vi "Append Block.vi"(10 "block in":u8[](array[numeric]) format="%02x", 11 "Hash Function in":refnum<class "NI_SHA-256.lvclass">) -> (3 "Hash Function out":refnum<class "NI_SHA-256.lvclass">)   [LabVIEW 2013, in "NI_SHA-256(2013).lvlib" / "NI_SHA-256.lvclass"]
uses:
  NI_SHA-256.lvclass
  NI_SHA-256.lvclass/NI_SHA-256.ctl
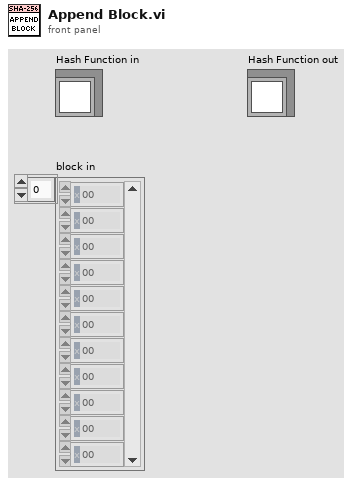
[diagram p1: front panel]
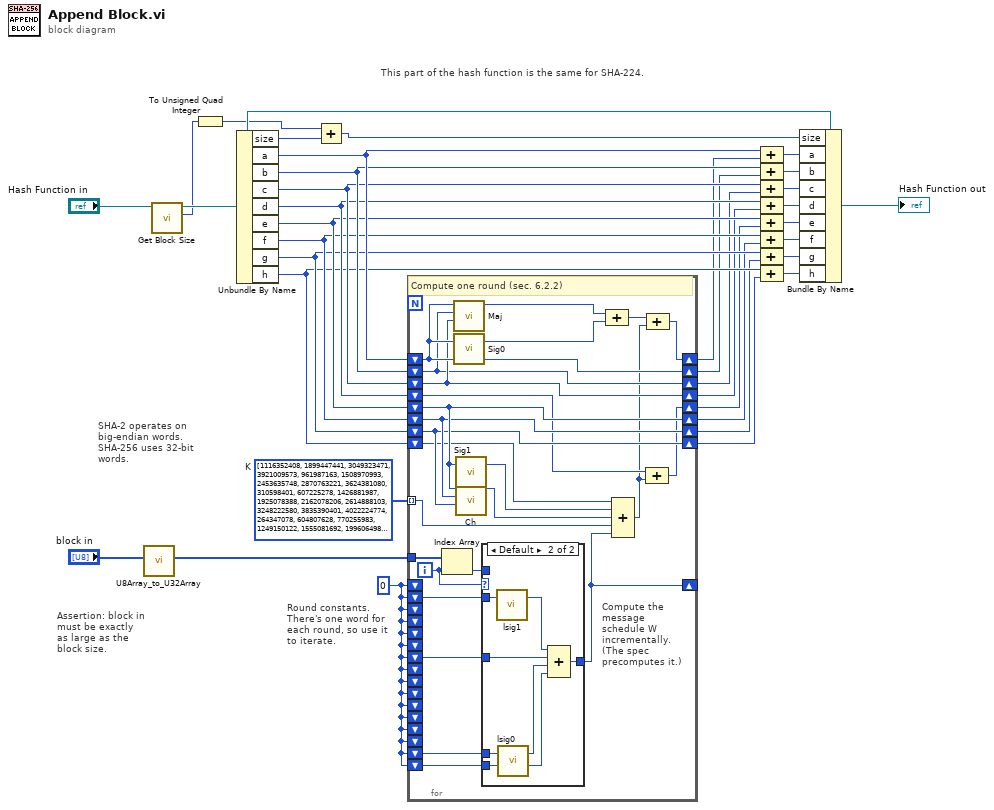
[diagram p0: block diagram]
diagram:
  w3 = u32 0
  w12 = u32[] [1116352408, 1899447441, 3049323471, 3921009573, 961987163, 1508970993, 2453635748, 2870763221, 3624381080, 310598401, 607225278, 1426881987, 1925078388, 2162078206, 2614888103, 3248222580, 3835390401, 4022224774, 264347078, 604807628, 770255983, 1249150122, 1555081692, 1996064986, 2554220882, 2821834349, 2952996808, 3210313671, 3336571891, 3584528711, 113926993, 338241895, 666307205, 773529912, 1294757372, 1396182291, 1695183700, 1986661051, 2177026350, 2456956037, 2730485921, 2820302411, 3259730800, 3345764771, 3516065817, 3600352804, 4094571909, 275423344, 430227734, 506948616, 659060556, 883997877, 958139571, 1322822218, 1537002063, 1747873779, 1955562222, 2024104815, 2227730452, 2361852424, 2428436474, 2756734187, 3204031479, 3329325298]  # K
  # "This part of the hash function is the same for SHA-224."
  # "Round constants. There's one word for each round, so use it to iterate."
  # "Assertion: block in must be exactly as large as the block size."
  # "SHA-2 operates on big-endian words. SHA-256 uses 32-bit words."
  n1 = call "U8Array_to_U32Array.vi"("U8"="block in") -> ("U32"=w1:u32[])  [unwired: 10 in]
  n2 = call "Get Block Size.vi"("Hash Function in"="Hash Function in") -> ("block size (bytes)"=w32:i32, "Hash Function out"=w33:refnum<class "NI_SHA-256.lvclass">)  [unwired: 9 in]
  n3 = To Unsigned Quad Integer(1:w32) -> (0:w31:u64)
  n4 = Unbundle By Name(w33) -> ("size"=w30:u64, "a"=w20:u32, "b"=w19:u32, "c"=w18:u32, "d"=w17:u32, "e"=w16:u32, "f"=w15:u32, "g"=w14:u32, "h"=w13:u32)
  n5 = Add(x=w31, y=w30) -> (x+y=w29:u64)
  n6 = for {
    shift-right: [w44] -> w11
    shift-left: w20 -> [w51]
    shift-right: [w51] -> w10
    shift-left: w19 -> [w49]
    shift-right: [w49] -> w9
    shift-left: w18 -> [w50]
    shift-right: [w50] -> w8
    shift-left: w17 -> [w53]
    shift-right: [w52] -> w7
    shift-left: w16 -> [w60]
    shift-right: [w60] -> w6
    shift-left: w15 -> [w59]
    shift-right: [w59] -> w5
    shift-left: w14 -> [w58]
    shift-right: [w58] -> w4
    shift-left: w13 -> [w57]
    tunnel: w12 -> [w54] mode=indexing
    tunnel: w1 -> [w43]
    shift-right: [w36] -> _
    shift-left: w3 -> [_]
    shift-left: w3 -> [w40]
    shift-left: w3 -> [_]
    shift-left: w3 -> [_]
    shift-left: w3 -> [_]
    shift-left: w3 -> [_]
    shift-left: w3 -> [w39]
    shift-left: w3 -> [_]
    shift-left: w3 -> [_]
    shift-left: w3 -> [_]
    shift-left: w3 -> [_]
    shift-left: w3 -> [_]
    shift-left: w3 -> [_]
    shift-left: w3 -> [_]
    shift-left: w3 -> [w38]
    shift-left: w3 -> [w37]
    i -> [w42]
    # "Compute the message schedule W incrementally. (The spec precomputes it.)"
    # "Compute one round (sec. 6.2.2)"
    n7 = Index Array(array=w43, index=w42) -> (element=w41:u32)
    n8 = call "Maj.vi"("z"=w50, "y"=w49, "x"=w51) -> ("Maj"=w48:u32)  [unwired: 8 in]
    n9 = call "Sig0.vi"("x"=w51) -> ("Sig0"=w47:u32)  [unwired: 2 in]
    n10 = call "Sig1.vi"("x"=w60) -> ("Sig1"=w56:u32)  [unwired: 2 in]
    n11 = call "Ch.vi"("z"=w58, "y"=w59, "x"=w60) -> ("Ch"=w55:u32)  [unwired: 8 in]
    n12 = case shown="Default" w42 {
      tunnel: w40 -> [_ w68]
      tunnel: w39 -> [_ w66]
      tunnel: w38 -> [_ w65]
      tunnel: w37 -> [_ w63]
      tunnel: [w61 w62] -> w36
      tunnel: w41 -> [w61 _]
      frame 0..15 {
      }
      frame Default {
        n13 = call "lsig1.vi"("x"=w68) -> ("lsig1"=w67:u32)  [unwired: 2 in]
        n14 = call "lsig0.vi"("x"=w65) -> ("lsig0"=w64:u32)  [unwired: 2 in]
        n15 = Compound Arithmetic op=ADD(w67, w66, w64, w63) -> (w62:u32)
      }
    }
    n16 = Compound Arithmetic op=ADD(w48, w47) -> (w46:u32)
    n17 = Compound Arithmetic op=ADD(w57, w56, w55, w54, w36) -> (w45:u32)
    n18 = Compound Arithmetic op=ADD(w53, w45) -> (w52:u32)
    n19 = Compound Arithmetic op=ADD(w46, w45) -> (w44:u32)
  }
  n20 = Compound Arithmetic op=ADD(w20, w11) -> (w28:u32)
  n21 = Compound Arithmetic op=ADD(w19, w10) -> (w27:u32)
  n22 = Compound Arithmetic op=ADD(w18, w9) -> (w26:u32)
  n23 = Compound Arithmetic op=ADD(w17, w8) -> (w25:u32)
  n24 = Compound Arithmetic op=ADD(w16, w7) -> (w24:u32)
  n25 = Compound Arithmetic op=ADD(w15, w6) -> (w23:u32)
  n26 = Compound Arithmetic op=ADD(w14, w5) -> (w22:u32)
  n27 = Compound Arithmetic op=ADD(w13, w4) -> (w21:u32)
  n28 = Bundle By Name(cluster=w33, "size"=w29, "a"=w28, "b"=w27, "c"=w26, "d"=w25, "e"=w24, "f"=w23, "g"=w22, "h"=w21) -> (→"Hash Function out":refnum<class "NI_SHA-256.lvclass">)
